vi "Get Database.vi"(8 "error in (no error)":errorcluster, 11 "Table Configuration in":refnum<class "Table Configuration.lvclass">) -> (0 "error out":errorcluster, 2 "Database":refnum<class "Database Interface.lvclass">, 3 "Table Configuration out":refnum<class "Table Configuration.lvclass">)   [LabVIEW 2020, in "Table.lvlib" / "Table Configuration.lvclass"]
uses:
  Table Configuration.lvclass
  Database Interfaces/Database Interface Class/Database Interface.lvclass
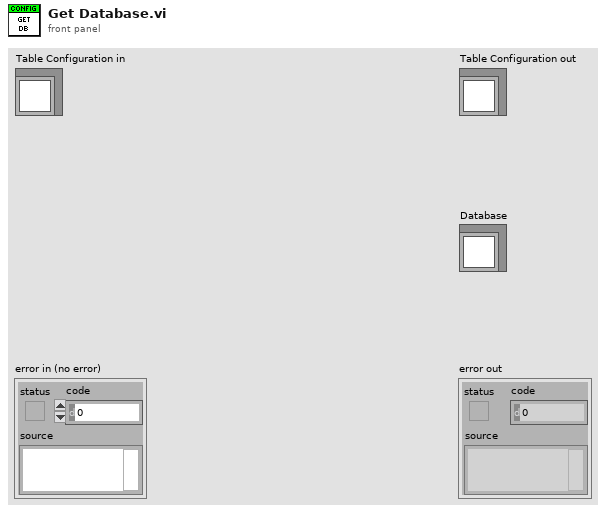
[diagram p1: front panel]
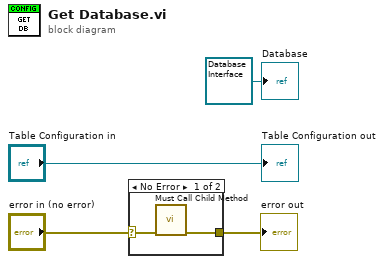
[diagram p0: block diagram]
diagram:
  n1 = case shown="No Error" "error in (no error)" {
    selector: "error in (no error)" -> [w6 w7]
    tunnel: [w5 w7] -> w2
    frame No Error {
      n2 = call "Must Call Child Method.vi"("error in"=w6) -> ("error out"=w5:errorcluster)  [unwired: 10 in]
    }
    frame Error {
    }
  }
  "error out" <- w2
  "Table Configuration out" <- "Table Configuration in"
  "Database" <- refnum<class "Database Interface.lvclass"> refnum ("Database")
